vi "solar_app Splash Update.vi"(8 "error in (no error)":errorcluster, 10 "Info":string, 11 "Splash VI Refnum in":refnum<vi>) -> (0 "error out":errorcluster, 3 "Splash VI Refnum out":refnum<vi>)   [LabVIEW 2018]
doc: "This updates the splash screen window information."
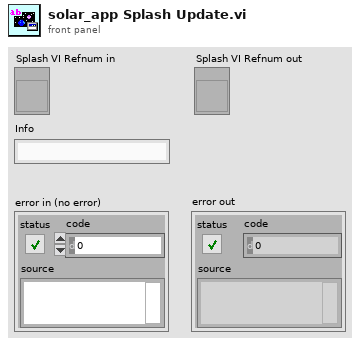
[diagram p1: front panel]
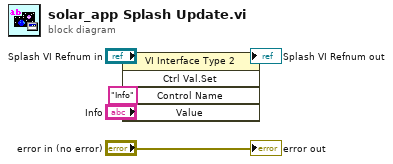
[diagram p0: block diagram]
diagram:
  n1 = invoke class="VI Interface Type 2" method="Ctrl Val.Set"(reference="Splash VI Refnum in", "Control Name"="Info", "Value"="Info") -> (reference out=→"Splash VI Refnum out":refnum<vi>)  [unwired: 2 in, 4 out]
  "error out" <- "error in (no error)"
